vi "in_diff and divided diff (dy over dx).vi"(9 "X":dbl[](array[numeric]), 11 "Y":dbl[](array[numeric]), 12 "i1":i32, 13 "i2":i32=-1) -> (10 "difference":dbl)   [LabVIEW 2020, in "NI_Gmath.lvlib"]
uses:
  NI_Gmath.lvlib
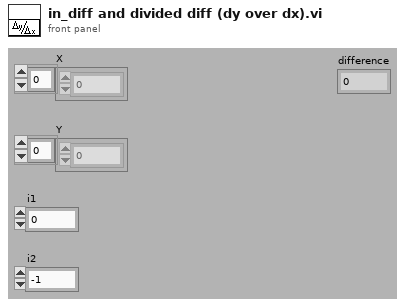
[diagram p1: front panel]
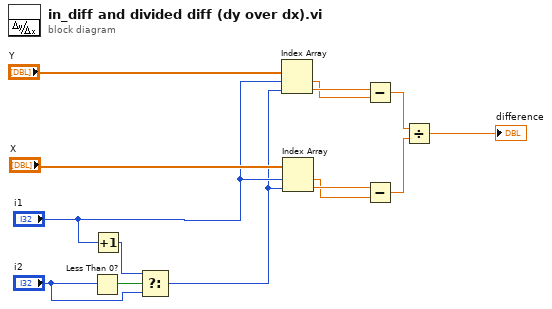
[diagram p0: block diagram]
diagram:
  n1 = Less Than 0?(x="i2") -> (x < 0?=w11:bool)
  n2 = Increment(x="i1") -> (x+1=w8:i32)
  n3 = Select(t=w8, s=w11, f="i2") -> (s? t:f=w7:i32)
  n4 = Index Array(array="Y", index #1="i1", index #2=w7) -> (element #1=w3:dbl, element #2=w4:dbl)
  n5 = Index Array(array="X", index #1="i1", index #2=w7) -> (element #1=w5:dbl, element #2=w6:dbl)
  n6 = Subtract(x=w4, y=w3) -> (x-y=w2:dbl)
  n7 = Subtract(x=w6, y=w5) -> (x-y=w1:dbl)
  n8 = Divide(x=w2, y=w1) -> (x/y=→"difference":dbl)
